vi "Execute.vi"(11 "Application in":refnum<class "Application.lvclass">) -> (0 "error out":errorcluster, 3 "Application out":refnum<class "Application.lvclass">)   [LabVIEW 2010, in "Application.lvclass"]
doc: "This VI MUST be overridden by child classes. Children should place their main execution logic in this VI. This VI will only be called if Setup does not return any errors."
uses:
  Application.lvclass
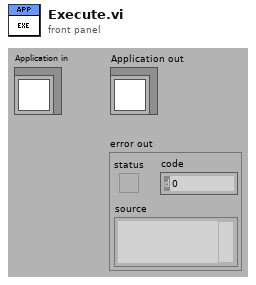
[diagram p1: front panel]
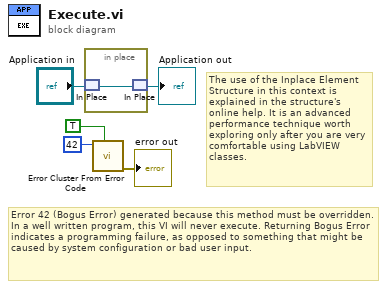
[diagram p0: block diagram]
diagram:
  # "The use of the Inplace Element Structure in this context is explained in the structure's online help. It is an advanced performance technique worth exploring only after you are very comfortable using LabVIEW classes."
  # "Error 42 (Bogus Error) generated because this method must be overridden. In a well written program, this VI will never execute. Returning Bogus Error indicates a programming failure, as opposed to something that might be caused by system configuration or bad user input."
  n1 = in-place {
    n2 = in-place-match #1("Application in") -> (w6:refnum<class "Application.lvclass">)
    n3 = in-place-match #1(w6) -> (→"Application out":refnum<class "Application.lvclass">)
  }
  n4 = call <vilib>:"Error Cluster From Error Code.vi"("show call chain? (False)"=TRUE, "error code (0)"=42) -> ("error out"=→"error out":errorcluster)  [unwired: 7 in]
